vi "Tacking Helper Helper - Starting Angle Test.vi"(6 "Waypoint Array In":T1[](array[typedef]) {"Point Type" items=["Drive", "Round Port", "Round Starboard", "Stay"]}, 9 "Starting Angle":dbl, 10 "Tests whether the while\nloop is on its first step":bool, 11 "Step Number\nof While Loop":i32) -> (3 "Boolean out":bool)   [LabVIEW 2011]
doc: "This vi determines whether or not to use the starting angle. True means use the starting angle to start the next jump, False means use the secondary.\n\nWhen there array size is 0, it is the first tack and the starting angle should definitely be used, so it returns true.\n\nFor every other iteration, the vi takes the last two waypoint entries, finds the angle between them, and tests it against the starting angle. If it is within 0.1 rad of the starting angle (just to eliminate any problems caused by computer rounding) then the vi returns True, which tells the outside vi to use the start angle for the next jump."
uses:
  0x2-OCU-Think Comm/0x2 Typedefs/ocuWaypoint.ctl
  0x2-OCU-Think Comm/0x2 Typedefs/waypointTypes.ctl
  2 Typedefs/UTM Location.ctl
  <vilib>/Analysis/coordinate.llb/Absolute Angle Difference (scalar).vi
  <vilib>/Analysis/coordinate.llb/Wrap Angle (scalar).vi
  <vilib>/Analysis/coordinate.llb/Set Angle Unit.vi
  <vilib>/Analysis/NI_AAL_Angle.lvlib
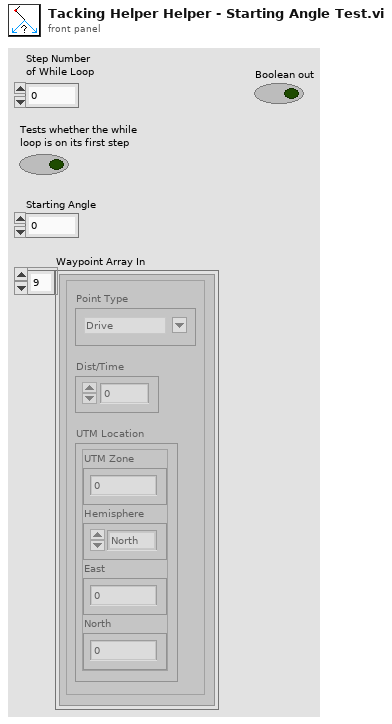
[diagram p1: front panel]
types:
  T1 = typedef "ocuWaypoint.ctl" = cluster{"Point Type":T2, "Dist/Time":dbl, "UTM Location":T3}
  T2 = typedef "waypointTypes.ctl" = u16
  T3 = typedef "UTM Location.ctl" = cluster{"UTM Zone":dbl, "Hemisphere":enum16{"North", "South"}, "East":dbl, "North":dbl}
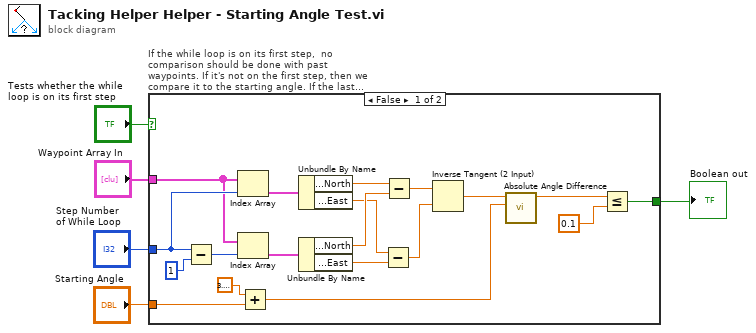
[diagram p0: block diagram]
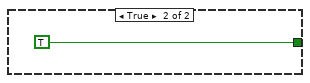
[diagram p2: hidden frame]
diagram:
  n1 = case "If the while loop is on its first step,  no comparison should be done with past waypoints. If it's not on the first step, then we compare it to the starting angle. If the last angle used was the starting angle, true is returned and we use the starting angle again next." shown="False" "Tests whether the while\nloop is on its first step" {
    tunnel: "Waypoint Array In" -> [w13 _]
    tunnel: "Step Number\nof While Loop" -> [w14 _]
    tunnel: "Starting Angle" -> [w8 _]
    tunnel: [w9 TRUE] -> w5
    frame False {
      n2 = Subtract(x=w14, y=1 ("x")) -> (x-y=w24:i32)
      n3 = Index Array(array=w13, index=w14) -> (element=w23:T1)
      n4 = Index Array(array=w13, index=w24) -> (element=w22:T1)
      n5 = Add(x=3.141592653589793, y=w8) -> (x+y=w6:dbl)
      n6 = Unbundle By Name(w23) -> ("UTM Location.North"=w20:dbl, "UTM Location.East"=w19:dbl)
      n7 = Unbundle By Name(w22) -> ("UTM Location.North"=w21:dbl, "UTM Location.East"=w18:dbl)
      n8 = Subtract(x=w19, y=w18) -> (x-y=w17:dbl)
      n9 = Subtract(x=w20, y=w21) -> (x-y=w16:dbl)
      n10 = Inverse Tangent (2 Input)(1:w17, 2:w16) -> (0:w12:dbl)
      n11 = call-poly <vilib>:"Absolute Angle Difference.vi"("angle 2"=w6, "angle 1"=w12) -> ("absolute angle difference"=w11:dbl)  [unwired: 8 in, 1 out]
      n12 = Less Or Equal?(x=w11, y=0.1) -> (x <= y?=w9:bool)
    }
    frame True {
    }
  }
  "Boolean out" <- w5
